vi "Keithley 622x Get Settings.vi"(8 "error in":errorcluster, 11 "VISA resource name":refnum<visa-resource-name>) -> (0 "error out":errorcluster, 1 "data string out":string, 2 "Settings":string[](array[string]), 3 "VISA resource name out":refnum<visa-resource-name>)   [LabVIEW 2021]
uses:
  GPIB/VISA  Send Receive.vi
  Simple VISA Reader/Simple VISA Reader Driver.lvclass
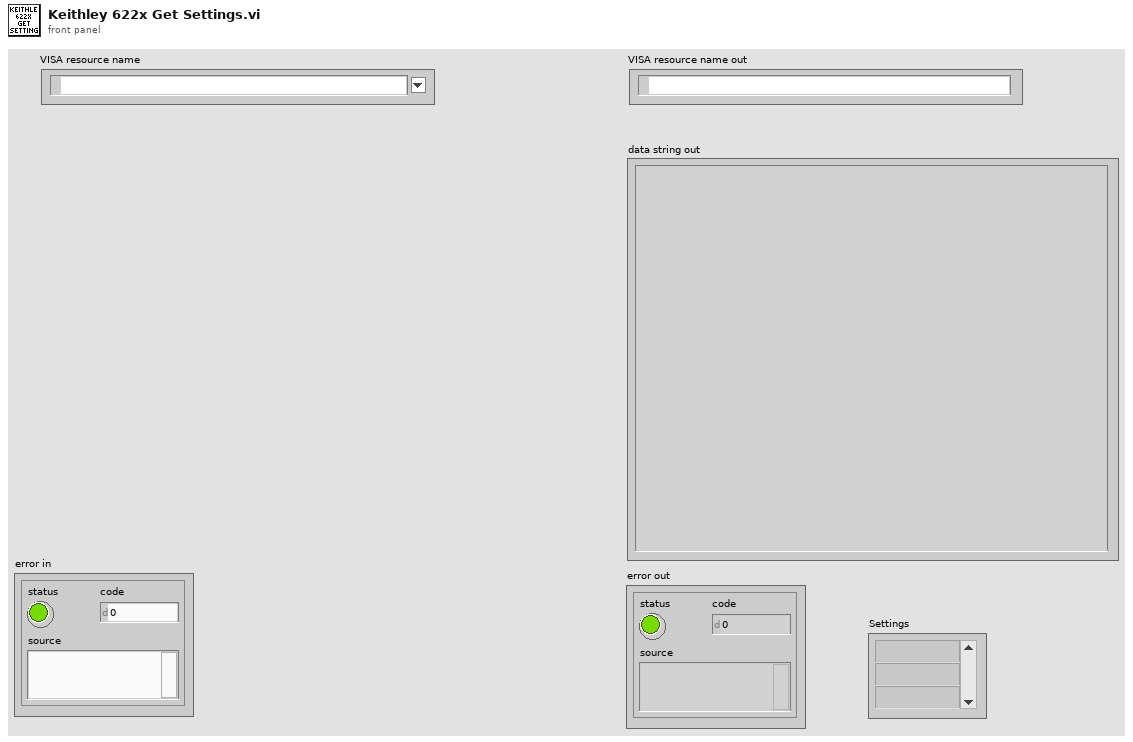
[diagram p1: front panel]
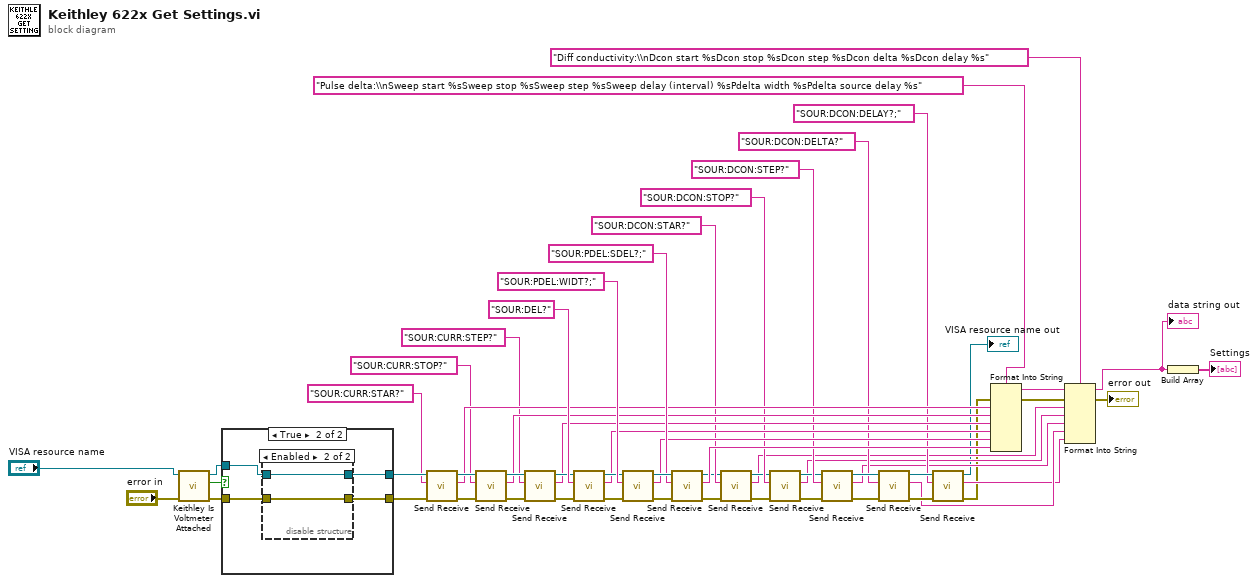
[diagram p0: block diagram]
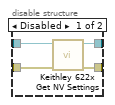
[diagram p3: hidden frame]
diagram:
  n1 = call "Keithley Is Voltmeter Attached.vi"("error in"="error in", "VISA resource name"="VISA resource name") -> ("error out"=w55:errorcluster, "Votmeter present"=w57:bool, "VISA resource name out"=w56:refnum<visa-resource-name>)  [unwired: 7 in]
  n2 = case shown="True" w57 {
    tunnel: w56 -> [w60 w64]
    tunnel: w55 -> [w59 w63]
    tunnel: [w59 w62] -> w28
    tunnel: [w60 w61] -> w38
    frame False {
    }
    frame True {
      n3 = disable-structure shown="Enabled" {
        disable-tunnel: w64 -> [w68 w70]
        disable-tunnel: w63 -> [w67 w69]
        disable-tunnel: [w66 w69] -> w62
        disable-tunnel: [w65 w70] -> w61
        frame Disabled {
          n4 = call "Keithley 622x Get NV Settings.vi"("error in"=w67, "VISA resource name"=w68) -> ("error out"=w66:errorcluster, "VISA resource name out"=w65:refnum<visa-resource-name>)  [unwired: 8 in]
        }
        frame Enabled {
        }
      }
    }
  }
  n5 = call-poly "Send Receive.vi"("error in (no error)"=w28, "data string in"="SOUR:CURR:STAR?", "VISA Resource Name"=w38) -> ("error out"=w42:errorcluster, "data string out"=w34:string, "VISA Resource Name Out"=w37:refnum<visa-resource-name>)  [unwired: 6 in]
  n6 = call-poly "Send Receive.vi"("error in (no error)"=w42, "data string in"="SOUR:CURR:STOP?", "VISA Resource Name"=w37) -> ("error out"=w41:errorcluster, "data string out"=w33:string, "VISA Resource Name Out"=w36:refnum<visa-resource-name>)  [unwired: 6 in]
  n7 = call-poly "Send Receive.vi"("error in (no error)"=w41, "data string in"="SOUR:CURR:STEP?", "VISA Resource Name"=w36) -> ("error out"=w40:errorcluster, "data string out"=w32:string, "VISA Resource Name Out"=w39:refnum<visa-resource-name>)  [unwired: 6 in]
  n8 = call-poly "Send Receive.vi"("error in (no error)"=w40, "data string in"="SOUR:DEL?", "VISA Resource Name"=w39) -> ("error out"=w44:errorcluster, "data string out"=w35:string, "VISA Resource Name Out"=w45:refnum<visa-resource-name>)  [unwired: 6 in]
  n9 = call-poly "Send Receive.vi"("error in (no error)"=w44, "data string in"="SOUR:PDEL:WIDT?;", "VISA Resource Name"=w45) -> ("error out"=w52:errorcluster, "data string out"=w47:string, "VISA Resource Name Out"=w51:refnum<visa-resource-name>)  [unwired: 6 in]
  n10 = call-poly "Send Receive.vi"("error in (no error)"=w52, "data string in"="SOUR:PDEL:SDEL?;", "VISA Resource Name"=w51) -> ("error out"=w12:errorcluster, "data string out"=w46:string, "VISA Resource Name Out"=w13:refnum<visa-resource-name>)  [unwired: 6 in]
  n11 = call-poly "Send Receive.vi"("error in (no error)"=w12, "data string in"="SOUR:DCON:STAR?", "VISA Resource Name"=w13) -> ("error out"=w18:errorcluster, "data string out"=w11:string, "VISA Resource Name Out"=w22:refnum<visa-resource-name>)  [unwired: 6 in]
  n12 = call-poly "Send Receive.vi"("error in (no error)"=w18, "data string in"="SOUR:DCON:STOP?", "VISA Resource Name"=w22) -> ("error out"=w19:errorcluster, "data string out"=w10:string, "VISA Resource Name Out"=w23:refnum<visa-resource-name>)  [unwired: 6 in]
  n13 = call-poly "Send Receive.vi"("error in (no error)"=w19, "data string in"="SOUR:DCON:STEP?", "VISA Resource Name"=w23) -> ("error out"=w20:errorcluster, "data string out"=w9:string, "VISA Resource Name Out"=w21:refnum<visa-resource-name>)  [unwired: 6 in]
  n14 = call-poly "Send Receive.vi"("error in (no error)"=w20, "data string in"="SOUR:DCON:DELTA?", "VISA Resource Name"=w21) -> ("error out"=w17:errorcluster, "data string out"=w8:string, "VISA Resource Name Out"=w16:refnum<visa-resource-name>)  [unwired: 6 in]
  n15 = call-poly "Send Receive.vi"("error in (no error)"=w17, "data string in"="SOUR:DCON:DELAY?;", "VISA Resource Name"=w16) -> ("error out"=w3:errorcluster, "data string out"=w7:string, "VISA Resource Name Out"=→"VISA resource name out":refnum<visa-resource-name>)  [unwired: 6 in]
  n16 = Format Into String(format string="Pulse delta:\\nSweep start %sSweep stop %sSweep step %sSweep delay (interval) %sPdelta width %sPdelta source delay %s", error in=w3, w34, w33, w32, w35, w47, w46) -> (resulting string=w6:string, error out=w4:errorcluster)  [unwired: 1 in]
  n17 = Format Into String(format string="Diff conductivity:\\nDcon start %sDcon stop %sDcon step %sDcon delta %sDcon delay %s", initial string=w6, error in=w4, w11, w10, w9, w8, w7) -> (resulting string=w5:string, error out=→"error out":errorcluster)
  "data string out" <- w5
  n18 = Build Array(w5) -> (→"Settings":string[])
